vi "UI Update Control Data By Name.vi"   [LabVIEW 2021]
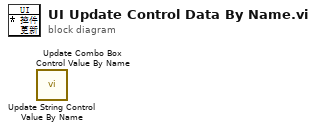
[diagram p0: block diagram]
diagram:
  n1 = call "Update String Control Value By Name.vi"() -> ()  [unwired: 9 in, 3 out]
  n2 = call "Update Combo Box Control Value By Name.vi"() -> ()  [unwired: 10 in, 2 out]
